vi "FindNodeCameFrom.vi"(1 "CameFrom":T1, 2 "nó atual":cluster{"id":dbl, "x":dbl, "y":dbl}) -> (8 "índice do nó atual":i32)   [LabVIEW 2016]
uses:
  CameFrom.ctl
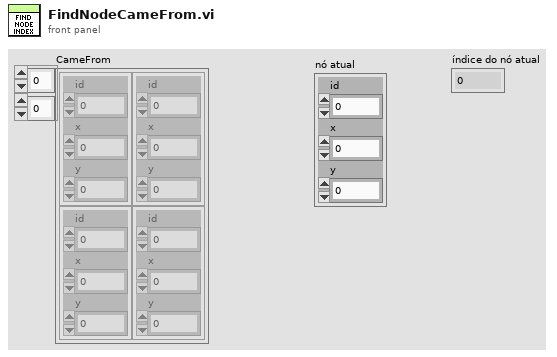
[diagram p1: front panel]
types:
  T1 = typedef "CameFrom.ctl" = cluster{"id":dbl, "x":dbl, "y":dbl}[][]
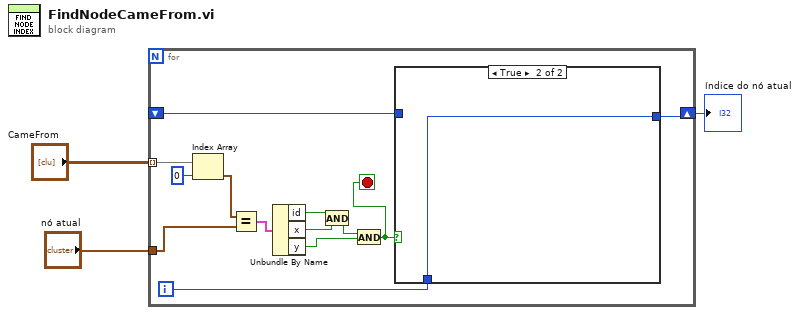
[diagram p0: block diagram]
diagram:
  n1 = for {
    tunnel: "CameFrom" -> [w16] mode=indexing
    tunnel: "nó atual" -> [w15]
    shift-right: [w6] -> w1
    shift-left: _ -> [w5]
    i -> [w7]
    stop <- w4 stop-if-true
    n2 = Index Array(array=w16, index=0) -> (element=w14:cluster{"id":dbl, "x":dbl, "y":dbl})
    n3 = Equal?(x=w14, y=w15) -> (x = y?=w12:cluster{"id":bool, "x":bool, "y":bool})
    n4 = Unbundle By Name(w12) -> ("id"=w11:bool, "x"=w10:bool, "y"=w8:bool)
    n5 = And(x=w11, y=w10) -> (x .and. y?=w9:bool)
    n6 = And(x=w9, y=w8) -> (x .and. y?=w4:bool)
    n7 = case shown="True" w4 {
      tunnel: w7 -> [_ w18]
      tunnel: [w17 w18] -> w6
      tunnel: w5 -> [w17 _]
      frame False {
      }
      frame True {
      }
    }
  }
  "índice do nó atual" <- w1
